vi "Auswahl fuer EKFG.vi"() -> ()   [LabVIEW 2020, in "AK-Schnittstelle.lvlib"]
uses:
  AK-Schnittstelle.lvlib
  Seiten/FT-IR/FGV FT-IR Gasliste Aktionen.ctl
  Visualisierungs Elemente/String - Ausgabefeld.ctl
  Seiten/FT-IR/FT-IR.lvlib
panel:
  in  "Alle Löschen":bool
  in  "Löschen":bool
  in  "Übernehmen":bool
  in  "Listenfeld 2":i32(listbox)
  in  "Stopp":bool
  out "Numerisch":dbl
  in  "Listenfeld":i32(listbox)
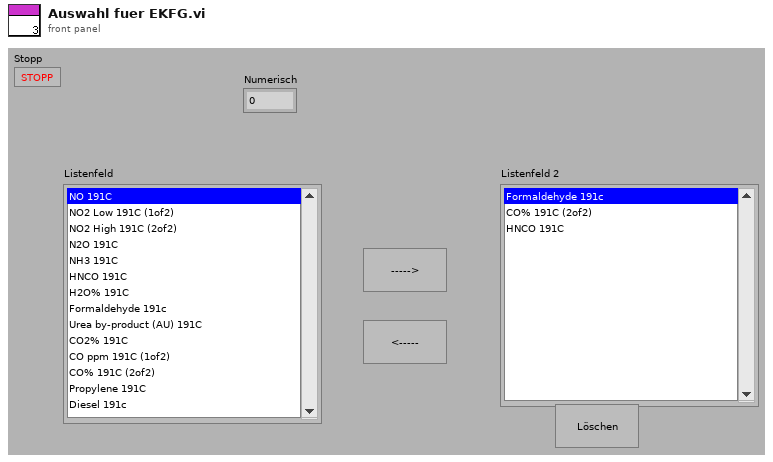
[diagram p1: front panel]
types:
  T1 = typedef "String - Ausgabefeld.ctl" = string
  T2 = typedef "FT-IR.lvlib/FGV FT-IR Gasliste Aktionen.ctl" = enum16{"lesen", "Gasliste FT-IR", "Gasliste ausgelesen", "laden", "speichern", "löschen"}
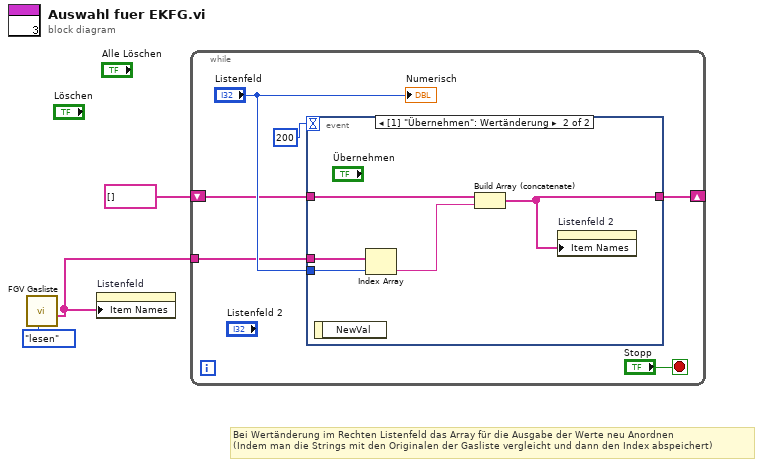
[diagram p0: block diagram]
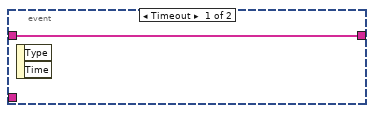
[diagram p2: hidden frame]
diagram:
  # "Bei Wertänderung im Rechten Listenfeld das Array für die Ausgabe der Werte neu Anordnen\n(Indem man die Strings mit den Originalen der Gasliste vergleicht und dann den Index abspeichert)"
  n1 = call "FGV Gasliste.vi"("Aktionen"=FGV_FT-IR_Gasliste_Aktionen."lesen") -> ("Aktuelle Gasliste gesamt"=w2:T1[])  [unwired: 8 in, 2 out]
  n2 = property on="Listenfeld" class="Listenfeld (strikt)"("Item Names"=w2) -> ()  [unwired: 2 in, 2 out]
  n3 = while {
    tunnel: w2 -> [w6]
    shift-right: [w4] -> _
    shift-left: T1[] [] ("Aktuelle Gasliste gesamt") -> [w5]
    stop <- "Stopp" stop-if-true
    n4 = event shown="[1] \"Übernehmen\": Wertänderung" {
      selector: _ -> [_ _]
      dyn-events: _ -> [_ _]
      timeout: 200 -> [_ _]
      tunnel: "Listenfeld" -> [_ w14]
      tunnel: w6 -> [_ w15]
      tunnel: w5 -> [w10 w13]
      tunnel: [w10 w11] -> w4
      event Timeout {
        n5 = event-data() -> ()  [unwired: 1 in, 2 out]
      }
      event "Übernehmen": Value Change {
        n6 = event-data() -> ()  [unwired: 1 in, 1 out]
        n7 = Index Array(array=w15, index=w14) -> (element=w12:T1)
        n8 = Build Array (concatenate)(w13, w12) -> (w11:T1[])
        n9 = property on="Listenfeld 2" class="Listenfeld (strikt)"("Item Names"=w11) -> ()  [unwired: 2 in, 2 out]
      }
    }
    "Numerisch" <- "Listenfeld"
  }
